vi "Calc Distance Matrix.vi"(11 "Coordinate[]":T1[](array[typedef])=[{"x"=38.24, "y"=20.42}, {"x"=39.57, "y"=26.15}, {"x"=40.56, "y"=25.32}, {"x"=36.26, "y"=23.12}, {"x"=33.48, "y"=10.54}, {"x"=37.56, "y"=12.19}, {"x"=38.42, "y"=13.11}, {"x"=37.52, "y"=20.44}, {"x"=41.23, "y"=9.1}, {"x"=41.17, "y"=13.05}, {"x"=36.08, "y"=-5.21}, {"x"=38.47, "y"=15.13}, {"x"=38.15, "y"=15.35}, {"x"=37.51, "y"=15.17}, {"x"=35.49, "y"=14.32}, {"x"=39.36, "y"=19.56}]) -> (3 "Distance Matrix":dbl[][](array[numeric]))   [LabVIEW 2015, in "TSP Library.lvlib"]
uses:
  TSP Library.lvlib
  TypeDef/Coordinate.ctl
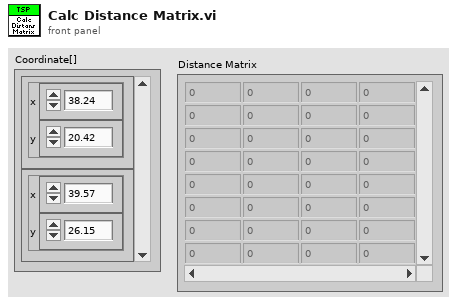
[diagram p1: front panel]
types:
  T1 = typedef "TSP Library.lvlib/Coordinate.ctl" = cluster{"x":dbl, "y":dbl}
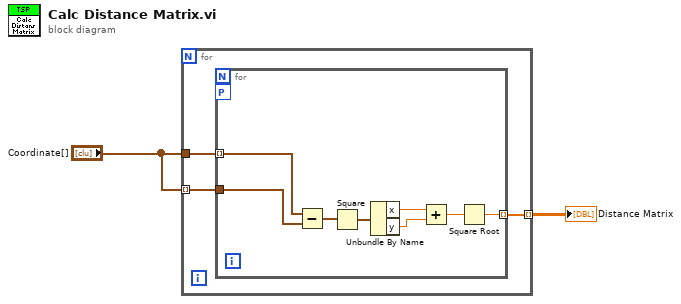
[diagram p0: block diagram]
diagram:
  n1 = for {
    tunnel: [w5] -> w2 mode=indexing
    tunnel: "Coordinate[]" -> [w4]
    tunnel: "Coordinate[]" -> [w3] mode=indexing
    n2 = for {
      tunnel: [w8] -> w5 mode=indexing
      tunnel: w4 -> [w7] mode=indexing
      tunnel: w3 -> [w6]
      workers-P: _ -> [_]
      n3 = Subtract(x=w7, y=w6) -> (x-y=w13:T1)
      n4 = Square(x=w13) -> (x^2=w12:T1)
      n5 = Unbundle By Name(w12) -> ("x"=w11:dbl, "y"=w10:dbl)
      n6 = Add(x=w11, y=w10) -> (x+y=w9:dbl)
      n7 = Square Root(x=w9) -> (sqrt(x)=w8:dbl)
    }
  }
  "Distance Matrix" <- w2
